vi "pf_Find_Property_Cluster.vi"(8 "error in (no error)":errorcluster, 9 "Properties Array":T1[](array[typedef])=[{"Name"="CameraName", "Type"=enum."PF_STRING", "Float.Min"=0.0, "Float.Max"=0.0, "Float.Value"=0.0, "Int.Min"=0, "Int.Max"=0, "Int.Value"=0, "String.Value"="MV-D1024E-3D01-160", "MODE.Values"=[], "MODE.Index"=0, "Flag"=enum."Undefined"}, {"Name"="DataOutMode", "Type"=enum."PF_MODE", "Float.Min"=0.0, "Float.Max"=0.0, "Float.Value"=0.0, "Int.Min"=0, "Int.Max"=0, "Int.Value"=0, "String.Value"="", "MODE.Values"=["Normal", "LFSR", "Ramp", "Lut"], "MODE.Index"=0, "Flag"=enum."Undefined"}, {"Name"="DataResolution", "Type"=enum."PF_MODE", "Float.Min"=0.0, "Float.Max"=0.0, "Float.Value"=0.0, "Int.Min"=0, "Int.Max"=0, "Int.Value"=0, "String.Value"="", "MODE.Values"=["Res12Bit", "Res10Bit", "Res8Bit"], "MODE.Index"=2, "Flag"=enum."Undefined"}, {"Name"="DigitalGain", "Type"=enum."PF_MODE", "Float.Min"=0.0, "Float.Max"=0.0, "Float.Value"=0.0, "Int.Min"=0, "Int.Max"=0, "Int.Value"=0, "String.Value"="", "MODE.Values"=["Gain1", "Gain2", "Gain4"], "MODE.Index"=0, "Flag"=enum."Undefined"}, {"Name"="EnStatusLine", "Type"=enum."PF_BOOL", "Float.Min"=0.0, "Float.Max"=0.0, "Float.Value"=0.0, "Int.Min"=0, "Int.Max"=0, "Int.Value"=0, "String.Value"="0", "MODE.Values"=[], "MODE.Index"=0, "Flag"=enum."Undefined"}, {"Name"="ExposureTime", "Type"=enum."PF_FLOAT", "Float.Min"=419.0, "Float.Max"=0.01, "Float.Value"=80.0, "Int.Min"=4294967295, "Int.Max"=4294967295, "Int.Value"=0, "String.Value"="80.000000", "MODE.Values"=[], "MODE.Index"=0, "Flag"=enum."Undefined"}, {"Name"="FactoryReset", "Type"=enum."PF_COMMAND", "Float.Min"=0.0, "Float.Max"=0.0, "Float.Value"=0.0, "Int.Min"=0, "Int.Max"=0, "Int.Value"=0, "String.Value"="", "MODE.Values"=[], "MODE.Index"=0, "Flag"=enum."Undefined"}, {"Name"="FrameRate", "Type"=enum."PF_STRING", "Float.Min"=0.0, "Float.Max"=0.0, "Float.Value"=0.0, "Int.Min"=0, "Int.Max"=0, "Int.Value"=0, "String.Value"="11.53", "MODE.Values"=[], "MODE.Index"=0, "Flag"=enum."Undefined"}, {"Name"="FrameTime", "Type"=enum."PF_FLOAT", "Float.Min"=419.0, "Float.Max"=0.01, "Float.Value"=86.7152, "Int.Min"=4294967295, "Int.Max"=4294967295, "Int.Value"=0, "String.Value"="86.715202", "MODE.Values"=[], "MODE.Index"=0, "Flag"=enum."Undefined"}, {"Name"="Reset", "Type"=enum."PF_COMMAND", "Float.Min"=0.0, "Float.Max"=0.0, "Float.Value"=0.0, "Int.Min"=0, "Int.Max"=0, "Int.Value"=0, "String.Value"="", "MODE.Values"=[], "MODE.Index"=0, "Flag"=enum."Undefined"}, {"Name"="Skim", "Type"=enum."PF_INT", "Float.Min"=-1.0, "Float.Max"=-1.0, "Float.Value"=0.0, "Int.Min"=8, "Int.Max"=0, "Int.Value"=0, "String.Value"="0", "MODE.Values"=[], "MODE.Index"=0, "Flag"=enum."Undefined"}, {"Name"="StoreDefaults", "Type"=enum."PF_COMMAND", "Float.Min"=0.0, "Float.Max"=0.0, "Float.Value"=0.0, "Int.Min"=0, "Int.Max"=0, "Int.Value"=0, "String.Value"="", "MODE.Values"=[], "MODE.Index"=0, "Flag"=enum."Undefined"}, {"Name"="Trigger.Source", "Type"=enum."PF_MODE", "Float.Min"=0.0, "Float.Max"=0.0, "Float.Value"=0.0, "Int.Min"=0, "Int.Max"=0, "Int.Value"=0, "String.Value"="", "MODE.Values"=["Free_Running", "Interface_Trigger", "IO_Trigger"], "MODE.Index"=0, "Flag"=enum."Undefined"}, {"Name"="Trigger.Invert", "Type"=enum."PF_BOOL", "Float.Min"=0.0, "Float.Max"=0.0, "Float.Value"=0.0, "Int.Min"=0, "Int.Max"=0, "Int.Value"=0, "String.Value"="0", "MODE.Values"=[], "MODE.Index"=0, "Flag"=enum."Undefined"}, {"Name"="Trigger.LevelControlled", "Type"=enum."PF_MODE", "Float.Min"=0.0, "Float.Max"=0.0, "Float.Value"=0.0, "Int.Min"=0, "Int.Max"=0, "Int.Value"=0, "String.Value"="", "MODE.Values"=["Software", "Trigger_Pulse_Width"], "MODE.Index"=0, "Flag"=enum."Undefined"}, {"Name"="Trigger.Delay", "Type"=enum."PF_FLOAT", "Float.Min"=419.0, "Float.Max"=0.0, "Float.Value"=0.0, "Int.Min"=4294967295, "Int.Max"=4294967295, "Int.Value"=0, "String.Value"="0.000000", "MODE.Values"=[], "MODE.Index"=0, "Flag"=enum."Undefined"}, {"Name"="Trigger.CFR", "Type"=enum."PF_BOOL", "Float.Min"=0.0, "Float.Max"=0.0, "Float.Value"=0.0, "Int.Min"=0, "Int.Max"=0, "Int.Value"=0, "String.Value"="0", "MODE.Values"=[], "MODE.Index"=0, "Flag"=enum."Undefined"}, {"Name"="Trigger.TriggerResolution", "Type"=enum."PF_INT", "Float.Min"=-1.0, "Float.Max"=-1.0, "Float.Value"=0.0, "Int.Min"=255, "Int.Max"=0, "Int.Value"=0, "String.Value"="0", "MODE.Values"=[], "MODE.Index"=0, "Flag"=enum."Undefined"}, {"Name"="Trigger.Interleave", "Type"=enum."PF_BOOL", "Float.Min"=0.0, "Float.Max"=0.0, "Float.Value"=0.0, "Int.Min"=0, "Int.Max"=0, "Int.Value"=0, "String.Value"="0", "MODE.Values"=[], "MODE.Index"=0, "Flag"=enum."Undefined"}, {"Name"="Counter.Image", "Type"=enum."PF_INT", "Float.Min"=-1.0, "Float.Max"=-1.0, "Float.Value"=0.0, "Int.Min"=16777215, "Int.Max"=0, "Int.Value"=203483, "String.Value"="203483", "MODE.Values"=[], "MODE.Index"=0, "Flag"=enum."Undefined"}, {"Name"="Counter.MissedTrigger", "Type"=enum."PF_INT", "Float.Min"=-1.0, "Float.Max"=-1.0, "Float.Value"=0.0, "Int.Min"=255, "Int.Max"=0, "Int.Value"=85, "String.Value"="85", "MODE.Values"=[], "MODE.Index"=0, "Flag"=enum."Undefined"}, {"Name"="Counter.Time", "Type"=enum."PF_INT", "Float.Min"=0.0, "Float.Max"=0.0, "Float.Value"=0.0, "Int.Min"=0, "Int.Max"=0, "Int.Value"=465187413, "String.Value"="465187413", "MODE.Values"=[], "MODE.Index"=0, "Flag"=enum."Undefined"}, {"Name"="Strobe.Delay", "Type"=enum."PF_FLOAT", "Float.Min"=419.0, "Float.Max"=0.0, "Float.Value"=0.0, "Int.Min"=4294967295, "Int.Max"=4294967295, "Int.Value"=0, "String.Value"="0.000000", "MODE.Values"=[], "MODE.Index"=0, "Flag"=enum."Undefined"}, {"Name"="Strobe.PulseWidth", "Type"=enum."PF_FLOAT", "Float.Min"=419.0, "Float.Max"=0.0, "Float.Value"=1.0, "Int.Min"=4294967295, "Int.Max"=4294967295, "Int.Value"=0, "String.Value"="1.000000", "MODE.Values"=[], "MODE.Index"=0, "Flag"=enum."Undefined"}, {"Name"="Strobe.Invert", "Type"=enum."PF_BOOL", "Float.Min"=0.0, "Float.Max"=0.0, "Float.Value"=0.0, "Int.Min"=0, "Int.Max"=0, "Int.Value"=0, "String.Value"="0", "MODE.Values"=[], "MODE.Index"=0, "Flag"=enum."Undefined"}, {"Name"="Window.X", "Type"=enum."PF_INT", "Float.Min"=-1.0, "Float.Max"=-1.0, "Float.Value"=0.0, "Int.Min"=1012, "Int.Max"=0, "Int.Value"=0, "String.Value"="0", "MODE.Values"=[], "MODE.Index"=0, "Flag"=enum."Undefined"}, {"Name"="Window.Y", "Type"=enum."PF_INT", "Float.Min"=-1.0, "Float.Max"=-1.0, "Float.Value"=0.0, "Int.Min"=1023, "Int.Max"=0, "Int.Value"=0, "String.Value"="0", "MODE.Values"=[], "MODE.Index"=0, "Flag"=enum."Undefined"}, {"Name"="Window.W", "Type"=enum."PF_INT", "Float.Min"=-1.0, "Float.Max"=-1.0, "Float.Value"=0.0, "Int.Min"=1024, "Int.Max"=12, "Int.Value"=1024, "String.Value"="1024", "MODE.Values"=[], "MODE.Index"=0, "Flag"=enum."Undefined"}, {"Name"="Window.H", "Type"=enum."PF_INT", "Float.Min"=-1.0, "Float.Max"=-1.0, "Float.Value"=0.0, "Int.Min"=1024, "Int.Max"=1, "Int.Value"=1024, "String.Value"="1024", "MODE.Values"=[], "MODE.Index"=0, "Flag"=enum."Undefined"}, {"Name"="Window.Max", "Type"=enum."PF_COMMAND", "Float.Min"=0.0, "Float.Max"=0.0, "Float.Value"=0.0, "Int.Min"=0, "Int.Max"=0, "Int.Value"=0, "String.Value"="", "MODE.Values"=[], "MODE.Index"=0, "Flag"=enum."Undefined"}, {"Name"="MROI.Enable", "Type"=enum."PF_BOOL", "Float.Min"=0.0, "Float.Max"=0.0, "Float.Value"=0.0, "Int.Min"=0, "Int.Max"=0, "Int.Value"=0, "String.Value"="0", "MODE.Values"=[], "MODE.Index"=0, "Flag"=enum."Undefined"}, {"Name"="MROI.Htot", "Type"=enum."PF_INT", "Float.Min"=0.0, "Float.Max"=0.0, "Float.Value"=0.0, "Int.Min"=0, "Int.Max"=0, "Int.Value"=1024, "String.Value"="1024", "MODE.Values"=[], "MODE.Index"=0, "Flag"=enum."Undefined"}, {"Name"="MROI.MROI0_Y", "Type"=enum."PF_INT", "Float.Min"=-1.0, "Float.Max"=-1.0, "Float.Value"=0.0, "Int.Min"=1023, "Int.Max"=0, "Int.Value"=0, "String.Value"="0", "MODE.Values"=[], "MODE.Index"=0, "Flag"=enum."Undefined"}, {"Name"="MROI.MROI0_H", "Type"=enum."PF_INT", "Float.Min"=-1.0, "Float.Max"=-1.0, "Float.Value"=0.0, "Int.Min"=1024, "Int.Max"=1, "Int.Value"=1024, "String.Value"="1024", "MODE.Values"=[], "MODE.Index"=0, "Flag"=enum."Undefined"}, {"Name"="MROI.MROI1_Y", "Type"=enum."PF_INT", "Float.Min"=-1.0, "Float.Max"=-1.0, "Float.Value"=0.0, "Int.Min"=1023, "Int.Max"=0, "Int.Value"=1023, "String.Value"="1023", "MODE.Values"=[], "MODE.Index"=0, "Flag"=enum."Undefined"}, {"Name"="MROI.MROI1_H", "Type"=enum."PF_INT", "Float.Min"=-1.0, "Float.Max"=-1.0, "Float.Value"=0.0, "Int.Min"=1024, "Int.Max"=1, "Int.Value"=1, "String.Value"="1", "MODE.Values"=[], "MODE.Index"=0, "Flag"=enum."Undefined"}, {"Name"="MROI.MROI2_Y", "Type"=enum."PF_INT", "Float.Min"=-1.0, "Float.Max"=-1.0, "Float.Value"=0.0, "Int.Min"=1023, "Int.Max"=0, "Int.Value"=1023, "String.Value"="1023", "MODE.Values"=[], "MODE.Index"=0, "Flag"=enum."Undefined"}, {"Name"="MROI.MROI2_H", "Type"=enum."PF_INT", "Float.Min"=-1.0, "Float.Max"=-1.0, "Float.Value"=0.0, "Int.Min"=1024, "Int.Max"=1, "Int.Value"=1, "String.Value"="1", "MODE.Values"=[], "MODE.Index"=0, "Flag"=enum."Undefined"}, {"Name"="MROI.MROI3_Y", "Type"=enum."PF_INT", "Float.Min"=-1.0, "Float.Max"=-1.0, "Float.Value"=0.0, "Int.Min"=1023, "Int.Max"=0, "Int.Value"=1023, "String.Value"="1023", "MODE.Values"=[], "MODE.Index"=0, "Flag"=enum."Undefined"}, {"Name"="MROI.MROI3_H", "Type"=enum."PF_INT", "Float.Min"=-1.0, "Float.Max"=-1.0, "Float.Value"=0.0, "Int.Min"=1024, "Int.Max"=1, "Int.Value"=1, "String.Value"="1", "MODE.Values"=[], "MODE.Index"=0, "Flag"=enum."Undefined"}, {"Name"="MROI.MROI4_Y", "Type"=enum."PF_INT", "Float.Min"=-1.0, "Float.Max"=-1.0, "Float.Value"=0.0, "Int.Min"=1023, "Int.Max"=0, "Int.Value"=1023, "String.Value"="1023", "MODE.Values"=[], "MODE.Index"=0, "Flag"=enum."Undefined"}, {"Name"="MROI.MROI4_H", "Type"=enum."PF_INT", "Float.Min"=-1.0, "Float.Max"=-1.0, "Float.Value"=0.0, "Int.Min"=1024, "Int.Max"=1, "Int.Value"=1, "String.Value"="1", "MODE.Values"=[], "MODE.Index"=0, "Flag"=enum."Undefined"}, {"Name"="MROI.MROI5_Y", "Type"=enum."PF_INT", "Float.Min"=-1.0, "Float.Max"=-1.0, "Float.Value"=0.0, "Int.Min"=1023, "Int.Max"=0, "Int.Value"=1023, "String.Value"="1023", "MODE.Values"=[], "MODE.Index"=0, "Flag"=enum."Undefined"}, {"Name"="MROI.MROI5_H", "Type"=enum."PF_INT", "Float.Min"=-1.0, "Float.Max"=-1.0, "Float.Value"=0.0, "Int.Min"=1024, "Int.Max"=1, "Int.Value"=1, "String.Value"="1", "MODE.Values"=[], "MODE.Index"=0, "Flag"=enum."Undefined"}, {"Name"="MROI.MROI6_Y", "Type"=enum."PF_INT", "Float.Min"=-1.0, "Float.Max"=-1.0, "Float.Value"=0.0, "Int.Min"=1023, "Int.Max"=0, "Int.Value"=1023, "String.Value"="1023", "MODE.Values"=[], "MODE.Index"=0, "Flag"=enum."Undefined"}, {"Name"="MROI.MROI6_H", "Type"=enum."PF_INT", "Float.Min"=-1.0, "Float.Max"=-1.0, "Float.Value"=0.0, "Int.Min"=1024, "Int.Max"=1, "Int.Value"=1, "String.Value"="1", "MODE.Values"=[], "MODE.Index"=0, "Flag"=enum."Undefined"}, {"Name"="MROI.MROI7_Y", "Type"=enum."PF_INT", "Float.Min"=-1.0, "Float.Max"=-1.0, "Float.Value"=0.0, "Int.Min"=1023, "Int.Max"=0, "Int.Value"=1023, "String.Value"="1023", "MODE.Values"=[], "MODE.Index"=0, "Flag"=enum."Undefined"}, {"Name"="MROI.MROI7_H", "Type"=enum."PF_INT", "Float.Min"=-1.0, "Float.Max"=-1.0, "Float.Value"=0.0, "Int.Min"=1024, "Int.Max"=1, "Int.Value"=1, "String.Value"="1", "MODE.Values"=[], "MODE.Index"=0, "Flag"=enum."Undefined"}, {"Name"="MROI.MROI8_Y", "Type"=enum."PF_INT", "Float.Min"=-1.0, "Float.Max"=-1.0, "Float.Value"=0.0, "Int.Min"=1023, "Int.Max"=0, "Int.Value"=1023, "String.Value"="1023", "MODE.Values"=[], "MODE.Index"=0, "Flag"=enum."Undefined"}, {"Name"="MROI.MROI8_H", "Type"=enum."PF_INT", "Float.Min"=-1.0, "Float.Max"=-1.0, "Float.Value"=0.0, "Int.Min"=1024, "Int.Max"=1, "Int.Value"=1, "String.Value"="1", "MODE.Values"=[], "MODE.Index"=0, "Flag"=enum."Undefined"}, {"Name"="MROI.MROI9_Y", "Type"=enum."PF_INT", "Float.Min"=-1.0, "Float.Max"=-1.0, "Float.Value"=0.0, "Int.Min"=1023, "Int.Max"=0, "Int.Value"=1023, "String.Value"="1023", "MODE.Values"=[], "MODE.Index"=0, "Flag"=enum."Undefined"}, {"Name"="MROI.MROI9_H", "Type"=enum."PF_INT", "Float.Min"=-1.0, "Float.Max"=-1.0, "Float.Value"=0.0, "Int.Min"=1024, "Int.Max"=1, "Int.Value"=1, "String.Value"="1", "MODE.Values"=[], "MODE.Index"=0, "Flag"=enum."Undefined"}, {"Name"="MROI.MROI10_Y", "Type"=enum."PF_INT", "Float.Min"=-1.0, "Float.Max"=-1.0, "Float.Value"=0.0, "Int.Min"=1023, "Int.Max"=0, "Int.Value"=1023, "String.Value"="1023", "MODE.Values"=[], "MODE.Index"=0, "Flag"=enum."Undefined"}, {"Name"="MROI.MROI10_H", "Type"=enum."PF_INT", "Float.Min"=-1.0, "Float.Max"=-1.0, "Float.Value"=0.0, "Int.Min"=1024, "Int.Max"=1, "Int.Value"=1, "String.Value"="1", "MODE.Values"=[], "MODE.Index"=0, "Flag"=enum."Undefined"}, {"Name"="MROI.MROI11_Y", "Type"=enum."PF_INT", "Float.Min"=-1.0, "Float.Max"=-1.0, "Float.Value"=0.0, "Int.Min"=1023, "Int.Max"=0, "Int.Value"=1023, "String.Value"="1023", "MODE.Values"=[], "MODE.Index"=0, "Flag"=enum."Undefined"}, {"Name"="MROI.MROI11_H", "Type"=enum."PF_INT", "Float.Min"=-1.0, "Float.Max"=-1.0, "Float.Value"=0.0, "Int.Min"=1024, "Int.Max"=1, "Int.Value"=1, "String.Value"="1", "MODE.Values"=[], "MODE.Index"=0, "Flag"=enum."Undefined"}, {"Name"="MROI.MROI12_Y", "Type"=enum."PF_INT", "Float.Min"=-1.0, "Float.Max"=-1.0, "Float.Value"=0.0, "Int.Min"=1023, "Int.Max"=0, "Int.Value"=1023, "String.Value"="1023", "MODE.Values"=[], "MODE.Index"=0, "Flag"=enum."Undefined"}, {"Name"="MROI.MROI12_H", "Type"=enum."PF_INT", "Float.Min"=-1.0, "Float.Max"=-1.0, "Float.Value"=0.0, "Int.Min"=1024, "Int.Max"=1, "Int.Value"=1, "String.Value"="1", "MODE.Values"=[], "MODE.Index"=0, "Flag"=enum."Undefined"}, {"Name"="MROI.MROI13_Y", "Type"=enum."PF_INT", "Float.Min"=-1.0, "Float.Max"=-1.0, "Float.Value"=0.0, "Int.Min"=1023, "Int.Max"=0, "Int.Value"=1023, "String.Value"="1023", "MODE.Values"=[], "MODE.Index"=0, "Flag"=enum."Undefined"}, {"Name"="MROI.MROI13_H", "Type"=enum."PF_INT", "Float.Min"=-1.0, "Float.Max"=-1.0, "Float.Value"=0.0, "Int.Min"=1024, "Int.Max"=1, "Int.Value"=1, "String.Value"="1", "MODE.Values"=[], "MODE.Index"=0, "Flag"=enum."Undefined"}, {"Name"="MROI.MROI14_Y", "Type"=enum."PF_INT", "Float.Min"=-1.0, "Float.Max"=-1.0, "Float.Value"=0.0, "Int.Min"=1023, "Int.Max"=0, "Int.Value"=1023, "String.Value"="1023", "MODE.Values"=[], "MODE.Index"=0, "Flag"=enum."Undefined"}, {"Name"="MROI.MROI14_H", "Type"=enum."PF_INT", "Float.Min"=-1.0, "Float.Max"=-1.0, "Float.Value"=0.0, "Int.Min"=1024, "Int.Max"=1, "Int.Value"=1, "String.Value"="1", "MODE.Values"=[], "MODE.Index"=0, "Flag"=enum."Undefined"}, {"Name"="MROI.MROI15_Y", "Type"=enum."PF_INT", "Float.Min"=-1.0, "Float.Max"=-1.0, "Float.Value"=0.0, "Int.Min"=1023, "Int.Max"=0, "Int.Value"=1023, "String.Value"="1023", "MODE.Values"=[], "MODE.Index"=0, "Flag"=enum."Undefined"}, {"Name"="MROI.MROI15_H", "Type"=enum."PF_INT", "Float.Min"=-1.0, "Float.Max"=-1.0, "Float.Value"=0.0, "Int.Min"=1024, "Int.Max"=1, "Int.Value"=1, "String.Value"="1", "MODE.Values"=[], "MODE.Index"=0, "Flag"=enum."Undefined"}, {"Name"="Decimation.Y", "Type"=enum."PF_INT", "Float.Min"=-1.0, "Float.Max"=-1.0, "Float.Value"=0.0, "Int.Min"=15, "Int.Max"=1, "Int.Value"=1, "String.Value"="1", "MODE.Values"=[], "MODE.Index"=0, "Flag"=enum."Undefined"}, {"Name"="LUT.Mode", "Type"=enum."PF_MODE", "Float.Min"=0.0, "Float.Max"=0.0, "Float.Value"=0.0, "Int.Min"=0, "Int.Max"=0, "Int.Value"=0, "String.Value"="", "MODE.Values"=["Gain", "Gamma"], "MODE.Index"=0, "Flag"=enum."Undefined"}, {"Name"="LUT.Address", "Type"=enum."PF_INT", "Float.Min"=-1.0, "Float.Max"=-1.0, "Float.Value"=0.0, "Int.Min"=1023, "Int.Max"=0, "Int.Value"=8, "String.Value"="8", "MODE.Values"=[], "MODE.Index"=0, "Flag"=enum."Undefined"}, {"Name"="LUT.Data", "Type"=enum."PF_INT", "Float.Min"=-1.0, "Float.Max"=-1.0, "Float.Value"=0.0, "Int.Min"=255, "Int.Max"=0, "Int.Value"=2, "String.Value"="2", "MODE.Values"=[], "MODE.Index"=0, "Flag"=enum."Undefined"}, {"Name"="LUT.Value", "Type"=enum."PF_FLOAT", "Float.Min"=4.0, "Float.Max"=0.4, "Float.Value"=1.0, "Int.Min"=4294967295, "Int.Max"=4294967295, "Int.Value"=0, "String.Value"="1.000000", "MODE.Values"=[], "MODE.Index"=0, "Flag"=enum."Undefined"}, {"Name"="LUT.FileRead1", "Type"=enum."PF_STRING", "Float.Min"=0.0, "Float.Max"=0.0, "Float.Value"=0.0, "Int.Min"=0, "Int.Max"=0, "Int.Value"=0, "String.Value"="", "MODE.Values"=[], "MODE.Index"=0, "Flag"=enum."Undefined"}, {"Name"="LUT.FileSave1", "Type"=enum."PF_STRING", "Float.Min"=0.0, "Float.Max"=0.0, "Float.Value"=0.0, "Int.Min"=0, "Int.Max"=0, "Int.Value"=0, "String.Value"="", "MODE.Values"=[], "MODE.Index"=0, "Flag"=enum."Undefined"}, {"Name"="LinLog.Mode", "Type"=enum."PF_MODE", "Float.Min"=0.0, "Float.Max"=0.0, "Float.Value"=0.0, "Int.Min"=0, "Int.Max"=0, "Int.Value"=0, "String.Value"="", "MODE.Values"=["Off", "Low_compression", "Normal_compression", "High_compression", "User_defined"], "MODE.Index"=2, "Flag"=enum."Undefined"}, {"Name"="LinLog.Value1", "Type"=enum."PF_INT", "Float.Min"=-1.0, "Float.Max"=-1.0, "Float.Value"=0.0, "Int.Min"=30, "Int.Max"=0, "Int.Value"=22, "String.Value"="22", "MODE.Values"=[], "MODE.Index"=0, "Flag"=enum."Undefined"}, {"Name"="LinLog.Value2", "Type"=enum."PF_INT", "Float.Min"=-1.0, "Float.Max"=-1.0, "Float.Value"=0.0, "Int.Min"=30, "Int.Max"=0, "Int.Value"=19, "String.Value"="19", "MODE.Values"=[], "MODE.Index"=0, "Flag"=enum."Undefined"}, {"Name"="LinLog.Time1", "Type"=enum."PF_INT", "Float.Min"=-1.0, "Float.Max"=-1.0, "Float.Value"=0.0, "Int.Min"=1000, "Int.Max"=0, "Int.Value"=850, "String.Value"="850", "MODE.Values"=[], "MODE.Index"=0, "Flag"=enum."Undefined"}, {"Name"="LinLog.Time2", "Type"=enum."PF_INT", "Float.Min"=-1.0, "Float.Max"=-1.0, "Float.Value"=0.0, "Int.Min"=1000, "Int.Max"=0, "Int.Value"=950, "String.Value"="950", "MODE.Values"=[], "MODE.Index"=0, "Flag"=enum."Undefined"}, {"Name"="Correction.Mode", "Type"=enum."PF_MODE", "Float.Min"=0.0, "Float.Max"=0.0, "Float.Value"=0.0, "Int.Min"=0, "Int.Max"=0, "Int.Value"=0, "String.Value"="", "MODE.Values"=["Off", "Offset", "OffsetHotpixel", "Hotpixel", "OffsetGain", "OffsetGainHotpixel", "BlackRefOut", "GreyRefOut"], "MODE.Index"=5, "Flag"=enum."Undefined"}, {"Name"="Correction.SetBlackRef", "Type"=enum."PF_COMMAND", "Float.Min"=0.0, "Float.Max"=0.0, "Float.Value"=0.0, "Int.Min"=0, "Int.Max"=0, "Int.Value"=0, "String.Value"="", "MODE.Values"=[], "MODE.Index"=0, "Flag"=enum."Undefined"}, {"Name"="Correction.SetGreyRef", "Type"=enum."PF_COMMAND", "Float.Min"=0.0, "Float.Max"=0.0, "Float.Value"=0.0, "Int.Min"=0, "Int.Max"=0, "Int.Value"=0, "String.Value"="", "MODE.Values"=[], "MODE.Index"=0, "Flag"=enum."Undefined"}, {"Name"="Correction.Calculate", "Type"=enum."PF_COMMAND", "Float.Min"=0.0, "Float.Max"=0.0, "Float.Value"=0.0, "Int.Min"=0, "Int.Max"=0, "Int.Value"=0, "String.Value"="", "MODE.Values"=[], "MODE.Index"=0, "Flag"=enum."Undefined"}, {"Name"="Correction.SaveToFlash", "Type"=enum."PF_COMMAND", "Float.Min"=0.0, "Float.Max"=0.0, "Float.Value"=0.0, "Int.Min"=0, "Int.Max"=0, "Int.Value"=0, "String.Value"="", "MODE.Values"=[], "MODE.Index"=0, "Flag"=enum."Undefined"}, {"Name"="Correction.ValidationBlack", "Type"=enum."PF_COMMAND", "Float.Min"=0.0, "Float.Max"=0.0, "Float.Value"=0.0, "Int.Min"=0, "Int.Max"=0, "Int.Value"=0, "String.Value"="", "MODE.Values"=[], "MODE.Index"=0, "Flag"=enum."Undefined"}, {"Name"="Correction.ValidationGrey", "Type"=enum."PF_COMMAND", "Float.Min"=0.0, "Float.Max"=0.0, "Float.Value"=0.0, "Int.Min"=0, "Int.Max"=0, "Int.Value"=0, "String.Value"="", "MODE.Values"=[], "MODE.Index"=0, "Flag"=enum."Undefined"}, {"Name"="Average.Value", "Type"=enum."PF_INT", "Float.Min"=-1.0, "Float.Max"=-1.0, "Float.Value"=0.0, "Int.Min"=4095, "Int.Max"=0, "Int.Value"=336, "String.Value"="336", "MODE.Values"=[], "MODE.Index"=0, "Flag"=enum."Undefined"}, {"Name"="Voltages.BlackLevelOffset", "Type"=enum."PF_INT", "Float.Min"=-1.0, "Float.Max"=-1.0, "Float.Value"=0.0, "Int.Min"=4095, "Int.Max"=0, "Int.Value"=3345, "String.Value"="3345", "MODE.Values"=[], "MODE.Index"=0, "Flag"=enum."Undefined"}, {"Name"="PeakDetector.Mode", "Type"=enum."PF_MODE", "Float.Min"=0.0, "Float.Max"=0.0, "Float.Value"=0.0, "Int.Min"=0, "Int.Max"=0, "Int.Value"=0, "String.Value"="", "MODE.Values"=["2D only", "2D and 3D", "3D only"], "MODE.Index"=1, "Flag"=enum."Undefined"}, {"Name"="PeakDetector.Threshold", "Type"=enum."PF_INT", "Float.Min"=-1.0, "Float.Max"=-1.0, "Float.Value"=0.0, "Int.Min"=4095, "Int.Max"=0, "Int.Value"=700, "String.Value"="700", "MODE.Values"=[], "MODE.Index"=0, "Flag"=enum."Undefined"}, {"Name"="Header.PixelClock", "Type"=enum."PF_INT", "Float.Min"=0.0, "Float.Max"=0.0, "Float.Value"=0.0, "Int.Min"=0, "Int.Max"=0, "Int.Value"=80000000, "String.Value"="80000000", "MODE.Values"=[], "MODE.Index"=0, "Flag"=enum."Undefined"}, {"Name"="Header.ResolutionX", "Type"=enum."PF_INT", "Float.Min"=0.0, "Float.Max"=0.0, "Float.Value"=0.0, "Int.Min"=0, "Int.Max"=0, "Int.Value"=1024, "String.Value"="1024", "MODE.Values"=[], "MODE.Index"=0, "Flag"=enum."Undefined"}, {"Name"="Header.ResolutionY", "Type"=enum."PF_INT", "Float.Min"=0.0, "Float.Max"=0.0, "Float.Value"=0.0, "Int.Min"=0, "Int.Max"=0, "Int.Value"=1024, "String.Value"="1024", "MODE.Values"=[], "MODE.Index"=0, "Flag"=enum."Undefined"}], 10 "Property Name":string, 11 "IMAQ Session in":refnum<k11>) -> (0 "error out":errorcluster, 1 "Property element":T1, 2 "Property Name out":string, 3 "IMAQ Session out":refnum<k11>, 4 "Property index":i32)   [LabVIEW 2025, in "Photonfocus_Toolkit.lvlib"]
uses:
  Photonfocus_Toolkit.lvlib
  _Private/Controls/pf_Property_Cluster.ctl
  _Private/Controls/pf_Property_Type.ctl
  _Private/Controls/pf_Property_Flag.ctl
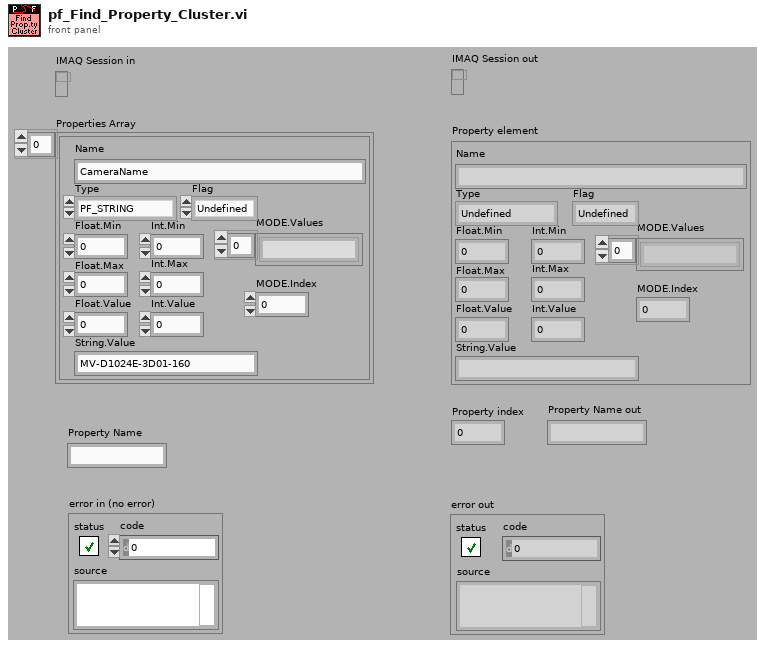
[diagram p1: front panel]
types:
  T1 = typedef "Photonfocus_Toolkit.lvlib/pf_Property_Cluster.ctl" = cluster{"Name":string, "Type":T2, "Float.Min":sgl, "Float.Max":sgl, "Float.Value":sgl, "Int.Min":u32, "Int.Max":u32, "Int.Value":u32, "String.Value":string, "MODE.Values":string[], "MODE.Index":i32, "Flag":T3}
  T2 = typedef "Photonfocus_Toolkit.lvlib/pf_Property_Type.ctl" = enum16{"Undefined", "PF_ROOT", "PF_INT", "PF_FLOAT", "PF_BOOL", "PF_MODE", "PF_REGISTER", "PF_STRING", "PF_BUFFER", "PF_STRUCT", "PF_ARRAY", "PF_COMMAND", "PF_EVENT"}
  T3 = typedef "Photonfocus_Toolkit.lvlib/pf_Property_Flag.ctl" = enum16{"Undefined", "RO", "WO", "RW"}
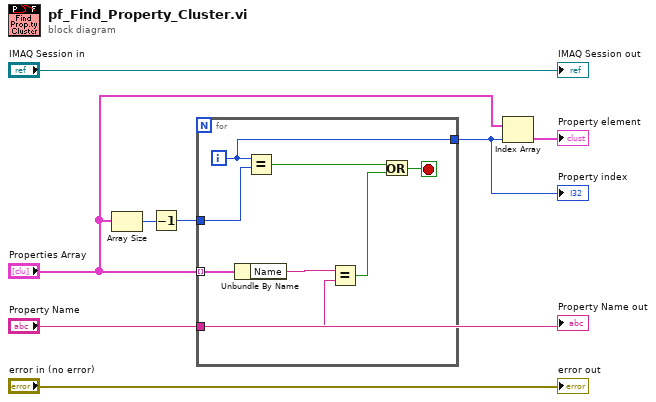
[diagram p0: block diagram]
diagram:
  n1 = Array Size(array="Properties Array") -> (size(s)=w8:i32)
  n2 = Decrement(x=w8) -> (x-1=w7:i32)
  n3 = for {
    tunnel: "Properties Array" -> [w16] mode=indexing
    tunnel: "Property Name" -> [w14]
    tunnel: w7 -> [w13]
    tunnel: [w10] -> w6
    i -> [w10]
    stop <- w9 stop-if-true
    n4 = Unbundle By Name(w16) -> ("Name"=w15:string)
    n5 = Equal?(x=w10, y=w13) -> (x = y?=w12:bool)
    n6 = Equal?(x=w15, y=w14) -> (x = y?=w11:bool)
    n7 = Or(x=w12, y=w11) -> (x .or. y?=w9:bool)
  }
  "Property index" <- w6
  n8 = Index Array(array="Properties Array", index=w6) -> (element=→"Property element":T1)
  "error out" <- "error in (no error)"
  "IMAQ Session out" <- "IMAQ Session in"
  "Property Name out" <- "Property Name"
